vi "HasVisited.vi"(8 "error in (no error)":errorcluster, 9 "Path":path, 11 "CVisitedSet in":refnum<class "CVisitedSet.lvclass">) -> (0 "error out":errorcluster, 1 "found?":bool, 3 "CVisitedSet out":refnum<class "CVisitedSet.lvclass">)   [LabVIEW 2020, in "DependencyInspection.lvlib" / "CVisitedSet.lvclass"]
uses:
  CVisitedSet.lvclass
  CVisitedSet.lvclass/CVisitedSet.ctl
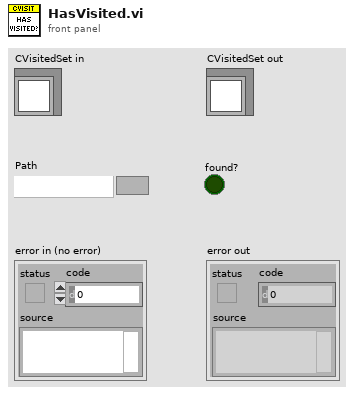
[diagram p1: front panel]
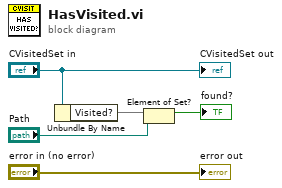
[diagram p0: block diagram]
diagram:
  n1 = Unbundle By Name("CVisitedSet in") -> ("Visited?"=w3:set{path})
  n2 = Element of Set?(10:"Path", 11:w3) -> (3:→"found?":bool)
  "error out" <- "error in (no error)"
  "CVisitedSet out" <- "CVisitedSet in"
